vi "check_if_cache_exists.vi"(8 "error in (no error)":errorcluster, 10 "Experiment Folder":path) -> (0 "error out":errorcluster, 2 "cache file out":path, 3 "exists":bool)   [LabVIEW 2016]
uses:
  <userlib>/_OpenG.lib/file/file.llb/File Exists - Scalar__ogtk.vi
panel:
  out "Experiment Name":string
  out "Device Folder Name":string
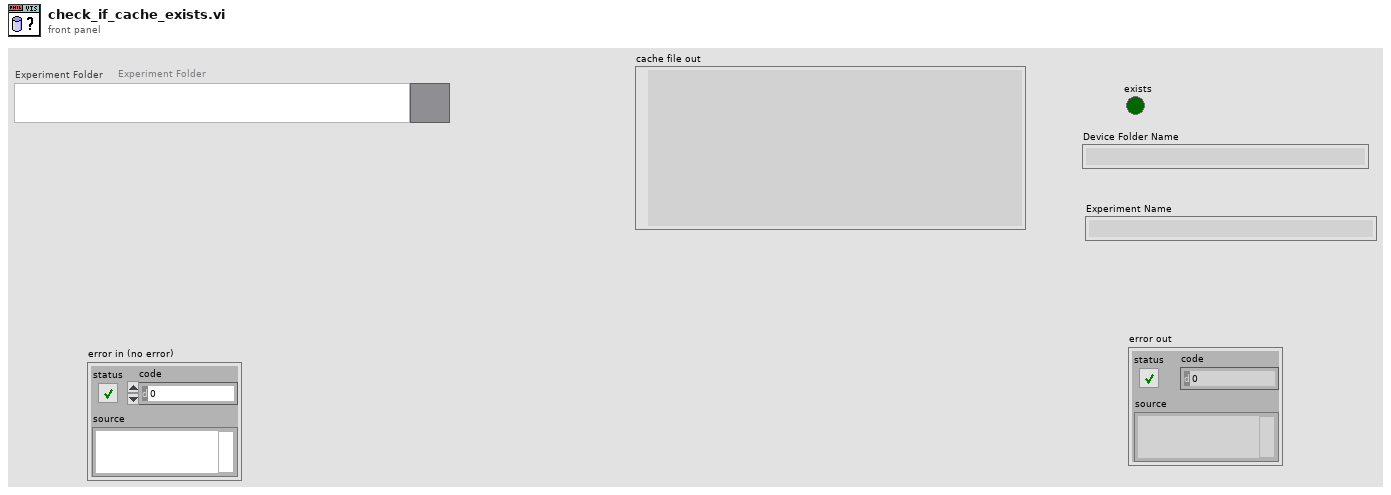
[diagram p1: front panel]
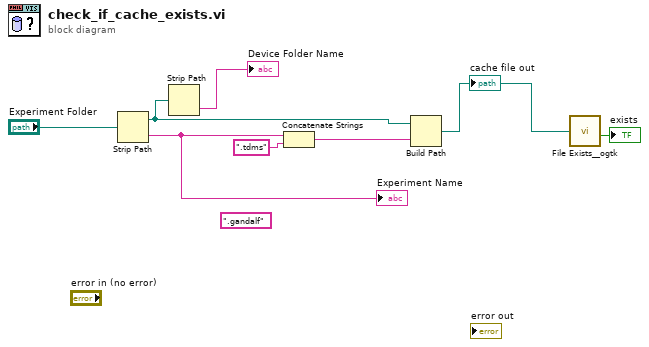
[diagram p0: block diagram]
diagram:
  (unwired) ".gandalf" ("string")
  n1 = Strip Path(path="Experiment Folder") -> (stripped path=w1:path, name=w5:string)
  "Experiment Name" <- w5
  n2 = Strip Path(path=w1) -> (name=→"Device Folder Name":string)  [unwired: 1 out]
  n3 = Concatenate Strings(w5, ".tdms" ("string")) -> (w4:string)
  n4 = Build Path(base path=w1, name or relative path=w4) -> (appended path=w3:path)
  "cache file out" <- w3
  n5 = call-poly <userlib>:"File Exists__ogtk.vi"("file path"=w3) -> ("exists"=→"exists":bool)  [unwired: 6 in, 1 out]
